vi "DSF.Simulation.Custom Device.Set Data Ref.vi"(8 "error in (no error)":errorcluster, 10 "Data Table Ref":T1, 11 "Simulated VeriStand Custom Device in":refnum<class "Simulated VeriStand Custom Device.lvclass">) -> (0 "error out":errorcluster, 3 "Simulated VeriStand Custom Device out":refnum<class "Simulated VeriStand Custom Device.lvclass">)   [LabVIEW 2016, in "Simulated VeriStand Custom Device.lvclass"]
uses:
  Simulated VeriStand Custom Device.lvclass
  <vilib>/NI Veristand/Custom Device API/Data Table Ref.ctl
  Simulated VeriStand Custom Device.lvclass/Simulated VeriStand Custom Device.ctl
  <vilib>/NI Veristand/Custom Device API/Custom Device API.lvlib
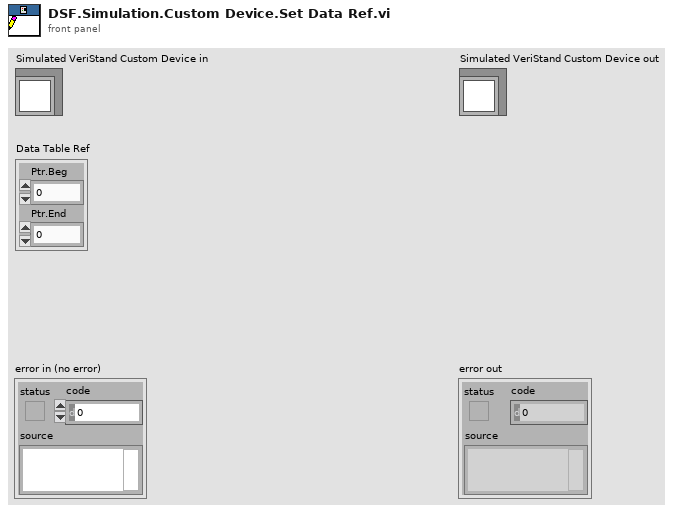
[diagram p1: front panel]
types:
  T1 = typedef "Custom Device API.lvlib/Data Table Ref.ctl" = cluster{"Ptr.Beg":u64, "Ptr.End":u64}
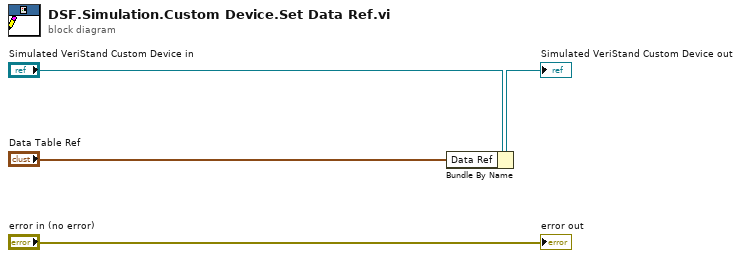
[diagram p0: block diagram]
diagram:
  n1 = Bundle By Name(cluster="Simulated VeriStand Custom Device in", "Data Ref"="Data Table Ref") -> (→"Simulated VeriStand Custom Device out":refnum<class "Simulated VeriStand Custom Device.lvclass">)
  "error out" <- "error in (no error)"
